vi "Read configuration.vi"(8 "error in":errorcluster, 11 "My System in":refnum<class "My System.lvclass">) -> (0 "error out":errorcluster, 2 "configuration":refnum<class "NISE_CEF_serializable configuration.lvclass">, 3 "My System out":refnum<class "My System.lvclass">)   [LabVIEW 2014, in "My System.lvclass"]
uses:
  My System.lvclass
  <vilib>/NI/Configuration Framework/serializable configuration/NISE_CEF_serializable configuration.lvclass
  My System.lvclass/My System.ctl
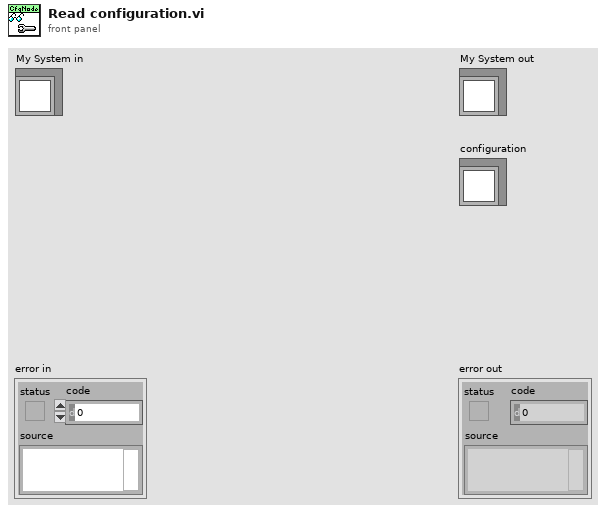
[diagram p1: front panel]
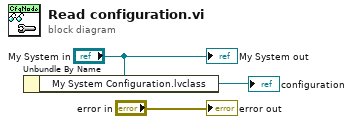
[diagram p0: block diagram]
diagram:
  n1 = Unbundle By Name("My System in") -> ("My System Configuration.lvclass"=→"configuration":refnum<class "My System Configuration.lvclass">)
  "error out" <- "error in"
  "My System out" <- "My System in"
